vi "Abstract_Function_Hierarchy.vi"   [LabVIEW 2021]
uses:
  One Terminal/Boolean/AbsFunc_One Term_Bool.lvclass
  One Terminal/STR/AbsFunc_One Term_STR.lvclass
  One Terminal/SGL/AbsFunc_One Term_SGL.lvclass
  One Terminal/DBL/AbsFunc_One Term_DBL.lvclass
  One Terminal/EXT/AbsFunc_One Term_EXT.lvclass
  One Terminal/Cmplx SGL/AbsFunc_One Term_Complex SGL.lvclass
  One Terminal/Cmplx DBL/AbsFunc_One Term_Complex DBL.lvclass
  One Terminal/Cmplx EXT/AbsFunc_One Term_Complex EXT.lvclass
  One Terminal/I8/AbsFunc_One Term_I8.lvclass
  One Terminal/I16/AbsFunc_One Term_I16.lvclass
  One Terminal/I32/AbsFunc_One Term_I32.lvclass
  One Terminal/I64/AbsFunc_One Term_I64.lvclass
  One Terminal/U8/AbsFunc_One Term_U8.lvclass
  One Terminal/U16/AbsFunc_One Term_U16.lvclass
  One Terminal/U32/AbsFunc_One Term_U32.lvclass
  One Terminal/U64/AbsFunc_One Term_U64.lvclass
  One Terminal/Time/AbsFunc_One Term_Time.lvclass
  One Terminal/WFM_Numeric/AbsFunc_One Term_WFM_Numeric.lvclass
  Two Terminal/Boolean/AbsFunc_Two Term_Bool.lvclass
  Two Terminal/STR/AbsFunc_Two Term_STR.lvclass
  Two Terminal/SGL/AbsFunc_Two Term_SGL.lvclass
  Two Terminal/EXT/AbsFunc_Two Term_EXT.lvclass
  Two Terminal/DBL/AbsFunc_Two Term_DBL.lvclass
  Two Terminal/Cmplx SGL/AbsFunc_Two Term_Complex SGL.lvclass
  Two Terminal/Cmplx DBL/AbsFunc_Two Term_Complex DBL.lvclass
  Two Terminal/Cmplx EXT/AbsFunc_Two Term_Complex EXT.lvclass
  Two Terminal/I8/AbsFunc_Two Term_I8.lvclass
  Two Terminal/I16/AbsFunc_Two Term_I16.lvclass
  Two Terminal/I32/AbsFunc_Two Term_I32.lvclass
  Two Terminal/I64/AbsFunc_Two Term_I64.lvclass
  Two Terminal/U8/AbsFunc_Two Term_U8.lvclass
  Two Terminal/U16/AbsFunc_Two Term_U16.lvclass
  Two Terminal/U32/AbsFunc_Two Term_U32.lvclass
  Two Terminal/U64/AbsFunc_Two Term_U64.lvclass
  Two Terminal/Time/AbsFunc_Two Term_Time.lvclass
  Two Terminal/WFM_Numeric/AbsFunc_Two Term_WFM_Numeric.lvclass
  Abs_Types/Boolean/Abs_Boolean.lvclass
  Abs_Types/String/Abs_String.lvclass
  Abs_Types/Single Float/Abs_Single Float.lvclass
  Abs_Types/Double Float/Abs_Double Float.lvclass
  Abs_Types/Extended Float/Abs_Extended Float.lvclass
  Abs_Types/Complex Single Float/Abs_Complex Single Float.lvclass
  Abs_Types/Complex Double Float/Abs_Complex Double Float.lvclass
  Abs_Types/Complex Extended Float/Abs_Complex Extended Float.lvclass
  Abs_Types/I8 Integer/Abs_I8 Integer.lvclass
  Abs_Types/I16 Integer/Abs_I16 Integer.lvclass
  Abs_Types/I32 Integer/Abs_I32 Integer.lvclass
  Abs_Types/I64 Integer/Abs_I64 Integer.lvclass
  Abs_Types/U8 Integer/Abs_U8 Integer.lvclass
  Abs_Types/U16 Integer/Abs_U16 Integer.lvclass
  Abs_Types/U32 Integer/Abs_U32 Integer.lvclass
  Abs_Types/U64 Integer/Abs_U64 Integer.lvclass
  Abs_Types/Time/Abs_Time.lvclass
  Abs_Types/Waveform/Abs_Waveform.lvclass
panel:
  # "SEE DIAGRAM\nFOR Hierarchy"
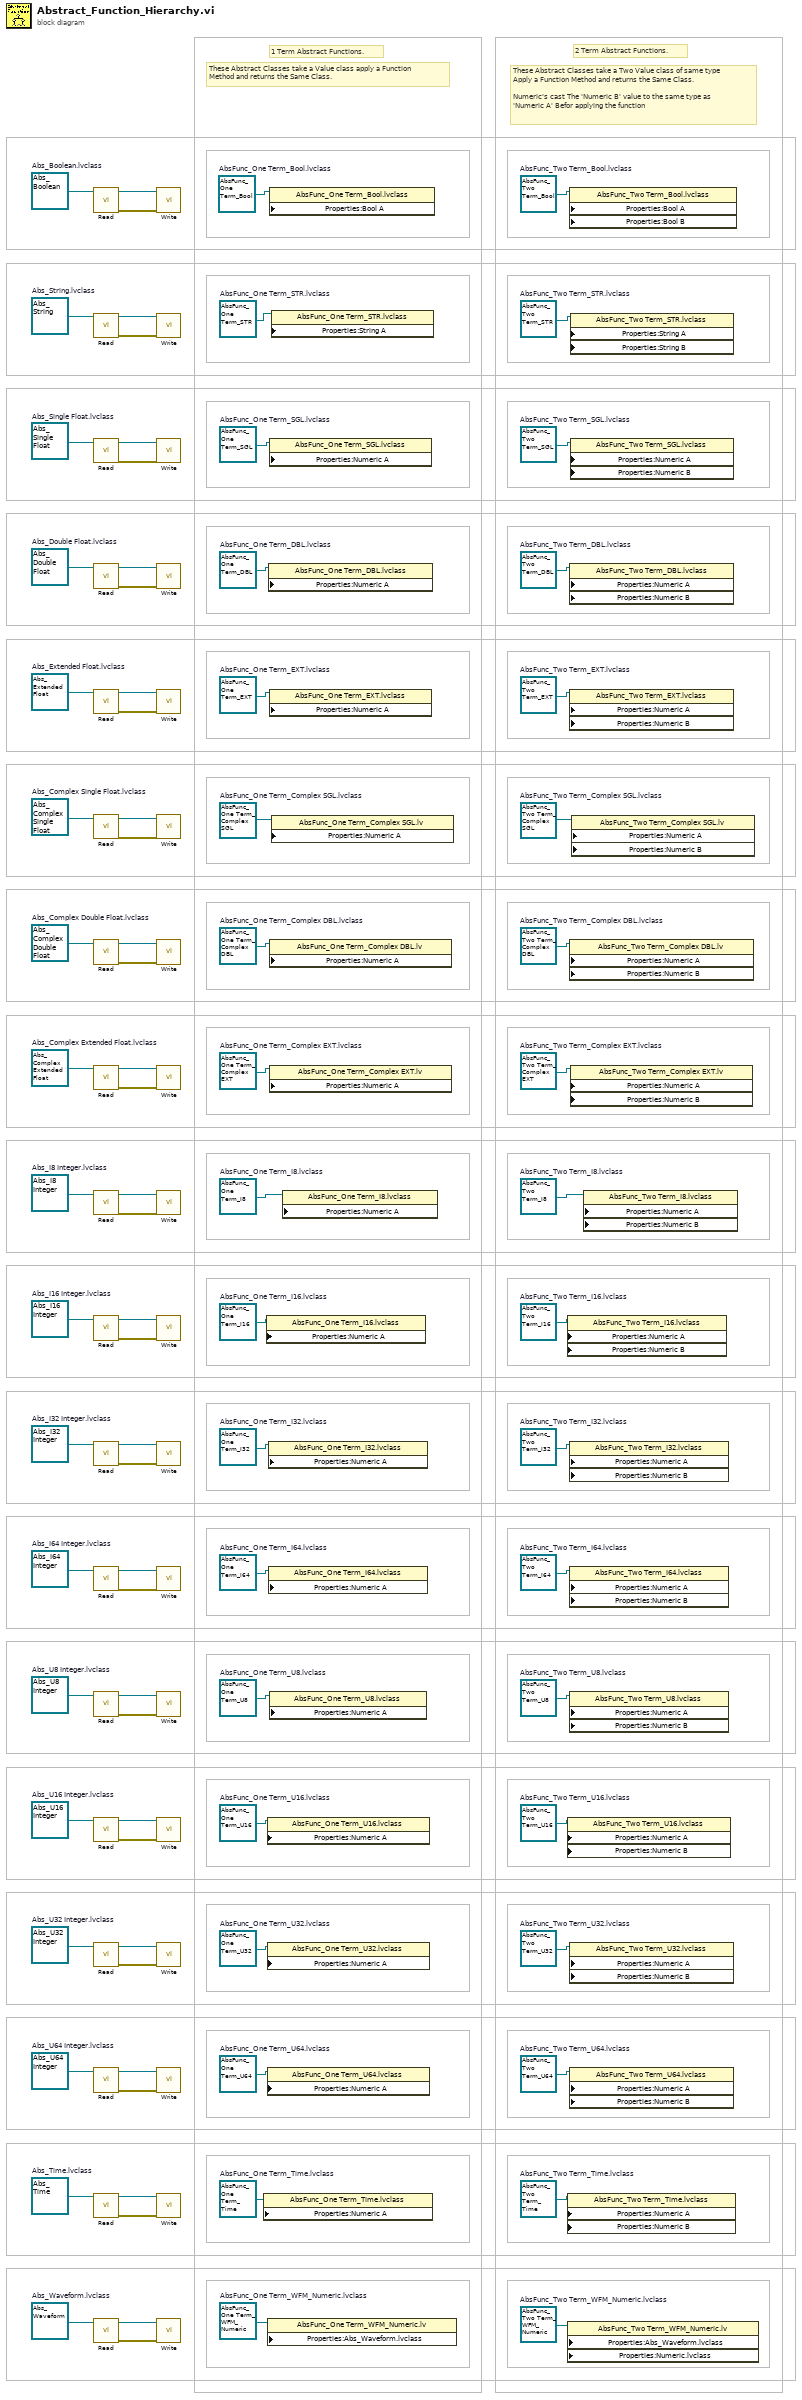
[diagram p0: block diagram]
diagram:
  w2 = refnum<class "Abs_Waveform.lvclass"> refnum  # Abs_Waveform.lvclass
  w7 = refnum<class "Abs_Time.lvclass"> refnum  # Abs_Time.lvclass
  w8 = refnum<class "Abs_U64 Integer.lvclass"> refnum  # Abs_U64 Integer.lvclass
  w11 = refnum<class "Abs_U32 Integer.lvclass"> refnum  # Abs_U32 Integer.lvclass
  w14 = refnum<class "Abs_U16 Integer.lvclass"> refnum  # Abs_U16 Integer.lvclass
  w17 = refnum<class "Abs_U8 Integer.lvclass"> refnum  # Abs_U8 Integer.lvclass
  w22 = refnum<class "Abs_I64 Integer.lvclass"> refnum  # Abs_I64 Integer.lvclass
  w23 = refnum<class "Abs_I32 Integer.lvclass"> refnum  # Abs_I32 Integer.lvclass
  w26 = refnum<class "Abs_I16 Integer.lvclass"> refnum  # Abs_I16 Integer.lvclass
  w29 = refnum<class "Abs_I8 Integer.lvclass"> refnum  # Abs_I8 Integer.lvclass
  w32 = refnum<class "Abs_Complex Extended Float.lvclass"> refnum  # Abs_Complex Extended Float.lvclass
  w35 = refnum<class "Abs_Complex Double Float.lvclass"> refnum  # Abs_Complex Double Float.lvclass
  w38 = refnum<class "Abs_Complex Single Float.lvclass"> refnum  # Abs_Complex Single Float.lvclass
  w41 = refnum<class "Abs_Extended Float.lvclass"> refnum  # Abs_Extended Float.lvclass
  w44 = refnum<class "Abs_Double Float.lvclass"> refnum  # Abs_Double Float.lvclass
  w47 = refnum<class "Abs_Single Float.lvclass"> refnum  # Abs_Single Float.lvclass
  w50 = refnum<class "Abs_String.lvclass"> refnum  # Abs_String.lvclass
  w55 = refnum<class "Abs_Boolean.lvclass"> refnum  # Abs_Boolean.lvclass
  w63 = refnum<class "AbsFunc_Two Term_WFM_Numeric.lvclass"> refnum  # AbsFunc_Two Term_WFM_Numeric.lvclass
  w64 = refnum<class "AbsFunc_Two Term_Time.lvclass"> refnum  # AbsFunc_Two Term_Time.lvclass
  w65 = refnum<class "AbsFunc_Two Term_U64.lvclass"> refnum  # AbsFunc_Two Term_U64.lvclass
  w66 = refnum<class "AbsFunc_Two Term_U32.lvclass"> refnum  # AbsFunc_Two Term_U32.lvclass
  w67 = refnum<class "AbsFunc_Two Term_U16.lvclass"> refnum  # AbsFunc_Two Term_U16.lvclass
  w68 = refnum<class "AbsFunc_Two Term_U8.lvclass"> refnum  # AbsFunc_Two Term_U8.lvclass
  w69 = refnum<class "AbsFunc_Two Term_I64.lvclass"> refnum  # AbsFunc_Two Term_I64.lvclass
  w70 = refnum<class "AbsFunc_Two Term_I32.lvclass"> refnum  # AbsFunc_Two Term_I32.lvclass
  w71 = refnum<class "AbsFunc_Two Term_I16.lvclass"> refnum  # AbsFunc_Two Term_I16.lvclass
  w72 = refnum<class "AbsFunc_Two Term_I8.lvclass"> refnum  # AbsFunc_Two Term_I8.lvclass
  w73 = refnum<class "AbsFunc_Two Term_Complex EXT.lvclass"> refnum  # AbsFunc_Two Term_Complex EXT.lvclass
  w74 = refnum<class "AbsFunc_Two Term_Complex DBL.lvclass"> refnum  # AbsFunc_Two Term_Complex DBL.lvclass
  w75 = refnum<class "AbsFunc_Two Term_Complex SGL.lvclass"> refnum  # AbsFunc_Two Term_Complex SGL.lvclass
  w77 = refnum<class "AbsFunc_Two Term_DBL.lvclass"> refnum  # AbsFunc_Two Term_DBL.lvclass
  w76 = refnum<class "AbsFunc_Two Term_EXT.lvclass"> refnum  # AbsFunc_Two Term_EXT.lvclass
  w78 = refnum<class "AbsFunc_Two Term_SGL.lvclass"> refnum  # AbsFunc_Two Term_SGL.lvclass
  w79 = refnum<class "AbsFunc_Two Term_STR.lvclass"> refnum  # AbsFunc_Two Term_STR.lvclass
  w80 = refnum<class "AbsFunc_Two Term_Bool.lvclass"> refnum  # AbsFunc_Two Term_Bool.lvclass
  w62 = refnum<class "AbsFunc_One Term_WFM_Numeric.lvclass"> refnum  # AbsFunc_One Term_WFM_Numeric.lvclass
  w61 = refnum<class "AbsFunc_One Term_Time.lvclass"> refnum  # AbsFunc_One Term_Time.lvclass
  w60 = refnum<class "AbsFunc_One Term_U64.lvclass"> refnum  # AbsFunc_One Term_U64.lvclass
  w59 = refnum<class "AbsFunc_One Term_U32.lvclass"> refnum  # AbsFunc_One Term_U32.lvclass
  w1 = refnum<class "AbsFunc_One Term_U16.lvclass"> refnum  # AbsFunc_One Term_U16.lvclass
  w58 = refnum<class "AbsFunc_One Term_U8.lvclass"> refnum  # AbsFunc_One Term_U8.lvclass
  w57 = refnum<class "AbsFunc_One Term_I64.lvclass"> refnum  # AbsFunc_One Term_I64.lvclass
  w56 = refnum<class "AbsFunc_One Term_I32.lvclass"> refnum  # AbsFunc_One Term_I32.lvclass
  w81 = refnum<class "AbsFunc_One Term_I16.lvclass"> refnum  # AbsFunc_One Term_I16.lvclass
  w82 = refnum<class "AbsFunc_One Term_I8.lvclass"> refnum  # AbsFunc_One Term_I8.lvclass
  w83 = refnum<class "AbsFunc_One Term_Complex EXT.lvclass"> refnum  # AbsFunc_One Term_Complex EXT.lvclass
  w84 = refnum<class "AbsFunc_One Term_Complex DBL.lvclass"> refnum  # AbsFunc_One Term_Complex DBL.lvclass
  w85 = refnum<class "AbsFunc_One Term_Complex SGL.lvclass"> refnum  # AbsFunc_One Term_Complex SGL.lvclass
  w86 = refnum<class "AbsFunc_One Term_EXT.lvclass"> refnum  # AbsFunc_One Term_EXT.lvclass
  w87 = refnum<class "AbsFunc_One Term_DBL.lvclass"> refnum  # AbsFunc_One Term_DBL.lvclass
  w88 = refnum<class "AbsFunc_One Term_SGL.lvclass"> refnum  # AbsFunc_One Term_SGL.lvclass
  w89 = refnum<class "AbsFunc_One Term_STR.lvclass"> refnum  # AbsFunc_One Term_STR.lvclass
  w90 = refnum<class "AbsFunc_One Term_Bool.lvclass"> refnum  # AbsFunc_One Term_Bool.lvclass
  # "1 Term Abstract Functions."
  # "These Abstract Classes take a Value class apply a Function \nMethod and returns the Same Class."
  # "These Abstract Classes take a Two Value class of same type\nApply a Function Method and returns the Same Class.\n\nNumeric's cast The 'Numeric B' value to the same type as \n'Numeric A' Befor applying the function"
  # "2 Term Abstract Functions."
  n1 = call-dynamic "Read.vi"("Boolean in"=w55) -> ("error out"=w54:errorcluster, "Boolean out"=w53:refnum<class "Abs_Boolean.lvclass">)  [unwired: 8 in, 1 out]
  n2 = call-dynamic "Read.vi"("Abs_String in"=w50) -> ("error out"=w52:errorcluster, "Abs_String out"=w51:refnum<class "Abs_String.lvclass">)  [unwired: 8 in, 1 out]
  n3 = call-dynamic "Read.vi"("Double Float.lvclass_340760 in"=w47) -> ("error out"=w49:errorcluster, "Double Float.lvclass_340760 out"=w48:refnum<class "Abs_Single Float.lvclass">)  [unwired: 8 in, 1 out]
  n4 = call-dynamic "Read.vi"("Double Float.lvclass_340760 in"=w44) -> ("error out"=w46:errorcluster, "Double Float.lvclass_340760 out"=w45:refnum<class "Abs_Double Float.lvclass">)  [unwired: 8 in, 1 out]
  n5 = call-dynamic "Read.vi"("Double Float.lvclass_340760 in"=w41) -> ("error out"=w43:errorcluster, "Double Float.lvclass_340760 out"=w42:refnum<class "Abs_Extended Float.lvclass">)  [unwired: 8 in, 1 out]
  n6 = call-dynamic "Read.vi"("Double Float.lvclass_340760 in"=w38) -> ("error out"=w40:errorcluster, "Double Float.lvclass_340760 out"=w39:refnum<class "Abs_Complex Single Float.lvclass">)  [unwired: 8 in, 1 out]
  n7 = call-dynamic "Read.vi"("Double Float.lvclass_340760 in"=w35) -> ("error out"=w37:errorcluster, "Double Float.lvclass_340760 out"=w36:refnum<class "Abs_Complex Double Float.lvclass">)  [unwired: 8 in, 1 out]
  n8 = call-dynamic "Read.vi"("Double Float.lvclass_340760 in"=w32) -> ("error out"=w34:errorcluster, "Double Float.lvclass_340760 out"=w33:refnum<class "Abs_Complex Extended Float.lvclass">)  [unwired: 8 in, 1 out]
  n9 = call-dynamic "Read.vi"("Double Float.lvclass_340760 in"=w29) -> ("error out"=w31:errorcluster, "Double Float.lvclass_340760 out"=w30:refnum<class "Abs_I8 Integer.lvclass">)  [unwired: 8 in, 1 out]
  n10 = call-dynamic "Read.vi"("Double Float.lvclass_340760 in"=w26) -> ("error out"=w28:errorcluster, "Double Float.lvclass_340760 out"=w27:refnum<class "Abs_I16 Integer.lvclass">)  [unwired: 8 in, 1 out]
  n11 = call-dynamic "Read.vi"("Double Float.lvclass_340760 in"=w23) -> ("error out"=w25:errorcluster, "Double Float.lvclass_340760 out"=w24:refnum<class "Abs_I32 Integer.lvclass">)  [unwired: 8 in, 1 out]
  n12 = call-dynamic "Read.vi"("Double Float.lvclass_340760 in"=w22) -> ("error out"=w21:errorcluster, "Double Float.lvclass_340760 out"=w20:refnum<class "Abs_I64 Integer.lvclass">)  [unwired: 8 in, 1 out]
  n13 = call-dynamic "Read.vi"("Double Float.lvclass_340760 in"=w17) -> ("error out"=w19:errorcluster, "Double Float.lvclass_340760 out"=w18:refnum<class "Abs_U8 Integer.lvclass">)  [unwired: 8 in, 1 out]
  n14 = call-dynamic "Read.vi"("Double Float.lvclass_340760 in"=w14) -> ("error out"=w16:errorcluster, "Double Float.lvclass_340760 out"=w15:refnum<class "Abs_U16 Integer.lvclass">)  [unwired: 8 in, 1 out]
  n15 = call-dynamic "Read.vi"("Double Float.lvclass_340760 in"=w11) -> ("error out"=w13:errorcluster, "Double Float.lvclass_340760 out"=w12:refnum<class "Abs_U32 Integer.lvclass">)  [unwired: 8 in, 1 out]
  n16 = call-dynamic "Read.vi"("Double Float.lvclass_340760 in"=w8) -> ("error out"=w10:errorcluster, "Double Float.lvclass_340760 out"=w9:refnum<class "Abs_U64 Integer.lvclass">)  [unwired: 8 in, 1 out]
  n17 = call-dynamic "Read.vi"("Double Float.lvclass_340760 in"=w7) -> ("error out"=w5:errorcluster, "Double Float.lvclass_340760 out"=w6:refnum<class "Abs_Time.lvclass">)  [unwired: 8 in, 1 out]
  n18 = call-dynamic "Read.vi"("Abs_Waveform in"=w2) -> ("error out"=w3:errorcluster, "Abs_Waveform out"=w4:refnum<class "Abs_Waveform.lvclass">)  [unwired: 8 in, 1 out]
  n19 = call-dynamic "Write.vi"("error in (no error)"=w54, "Boolean in"=w53) -> ()  [unwired: 8 in, 2 out]
  n20 = call-dynamic "Write.vi"("error in (no error)"=w52, "Abs_String in"=w51) -> ()  [unwired: 8 in, 2 out]
  n21 = call-dynamic "Write.vi"("error in (no error)"=w49, "Double Float.lvclass_340760 in"=w48) -> ()  [unwired: 8 in, 2 out]
  n22 = call-dynamic "Write.vi"("error in (no error)"=w46, "Double Float.lvclass in"=w45) -> ()  [unwired: 8 in, 2 out]
  n23 = call-dynamic "Write.vi"("error in (no error)"=w43, "Double Float.lvclass_340760 in"=w42) -> ()  [unwired: 8 in, 2 out]
  n24 = call-dynamic "Write.vi"("error in (no error)"=w40, "Double Float.lvclass_340760 in"=w39) -> ()  [unwired: 8 in, 2 out]
  n25 = call-dynamic "Write.vi"("error in (no error)"=w37, "Double Float.lvclass_340760 in"=w36) -> ()  [unwired: 8 in, 2 out]
  n26 = call-dynamic "Write.vi"("error in (no error)"=w34, "Double Float.lvclass_340760 in"=w33) -> ()  [unwired: 8 in, 2 out]
  n27 = call-dynamic "Write.vi"("error in (no error)"=w31, "Double Float.lvclass_340760 in"=w30) -> ()  [unwired: 8 in, 2 out]
  n28 = call-dynamic "Write.vi"("error in (no error)"=w28, "Double Float.lvclass_340760 in"=w27) -> ()  [unwired: 8 in, 2 out]
  n29 = call-dynamic "Write.vi"("error in (no error)"=w25, "Double Float.lvclass_340760 in"=w24) -> ()  [unwired: 8 in, 2 out]
  n30 = call-dynamic "Write.vi"("error in (no error)"=w21, "Double Float.lvclass_340760 in"=w20) -> ()  [unwired: 8 in, 2 out]
  n31 = call-dynamic "Write.vi"("error in (no error)"=w19, "Double Float.lvclass_340760 in"=w18) -> ()  [unwired: 8 in, 2 out]
  n32 = call-dynamic "Write.vi"("error in (no error)"=w16, "Double Float.lvclass_340760 in"=w15) -> ()  [unwired: 8 in, 2 out]
  n33 = call-dynamic "Write.vi"("error in (no error)"=w13, "Double Float.lvclass_340760 in"=w12) -> ()  [unwired: 8 in, 2 out]
  n34 = call-dynamic "Write.vi"("error in (no error)"=w10, "Double Float.lvclass_340760 in"=w9) -> ()  [unwired: 8 in, 2 out]
  n35 = call-dynamic "Write.vi"("error in (no error)"=w5, "Double Float.lvclass_340760 in"=w6) -> ()  [unwired: 8 in, 2 out]
  n36 = call-dynamic "Write.vi"("error in (no error)"=w3, "Abs_Waveform in"=w4) -> ()  [unwired: 8 in, 2 out]
  n37 = property class="AbsFunc_One Term_Time.lvclass" props=["Properties:Numeric A"](reference=w61) -> ()  [unwired: 2 in, 2 out]
  n38 = property class="AbsFunc_One Term_I16.lvclass" props=["Properties:Numeric A"](reference=w81) -> ()  [unwired: 2 in, 2 out]
  n39 = property class="AbsFunc_One Term_U16.lvclass" props=["Properties:Numeric A"](reference=w1) -> ()  [unwired: 2 in, 2 out]
  n40 = property class="AbsFunc_One Term_U32.lvclass" props=["Properties:Numeric A"](reference=w59) -> ()  [unwired: 2 in, 2 out]
  n41 = property class="AbsFunc_One Term_U64.lvclass" props=["Properties:Numeric A"](reference=w60) -> ()  [unwired: 2 in, 2 out]
  n42 = property class="AbsFunc_One Term_WFM_Numeric.lv" props=["Properties:Abs_Waveform.lvclass"](reference=w62) -> ()  [unwired: 2 in, 2 out]
  n43 = property class="AbsFunc_One Term_DBL.lvclass" props=["Properties:Numeric A"](reference=w87) -> ()  [unwired: 2 in, 2 out]
  n44 = property class="AbsFunc_One Term_I32.lvclass" props=["Properties:Numeric A"](reference=w56) -> ()  [unwired: 2 in, 2 out]
  n45 = property class="AbsFunc_One Term_I64.lvclass" props=["Properties:Numeric A"](reference=w57) -> ()  [unwired: 2 in, 2 out]
  n46 = property class="AbsFunc_One Term_Bool.lvclass" props=["Properties:Bool A"](reference=w90) -> ()  [unwired: 2 in, 2 out]
  n47 = property class="AbsFunc_One Term_SGL.lvclass" props=["Properties:Numeric A"](reference=w88) -> ()  [unwired: 2 in, 2 out]
  n48 = property class="AbsFunc_One Term_EXT.lvclass" props=["Properties:Numeric A"](reference=w86) -> ()  [unwired: 2 in, 2 out]
  n49 = property class="AbsFunc_One Term_Complex DBL.lv" props=["Properties:Numeric A"](reference=w84) -> ()  [unwired: 2 in, 2 out]
  n50 = property class="AbsFunc_One Term_Complex EXT.lv" props=["Properties:Numeric A"](reference=w83) -> ()  [unwired: 2 in, 2 out]
  n51 = property class="AbsFunc_One Term_U8.lvclass" props=["Properties:Numeric A"](reference=w58) -> ()  [unwired: 2 in, 2 out]
  n52 = property class="AbsFunc_One Term_STR.lvclass" props=["Properties:String A"](reference=w89) -> ()  [unwired: 2 in, 2 out]
  n53 = property class="AbsFunc_One Term_Complex SGL.lv" props=["Properties:Numeric A"](reference=w85) -> ()  [unwired: 2 in, 2 out]
  n54 = property class="AbsFunc_One Term_I8.lvclass" props=["Properties:Numeric A"](reference=w82) -> ()  [unwired: 2 in, 2 out]
  n55 = property class="AbsFunc_Two Term_I16.lvclass" props=["Properties:Numeric A", "Properties:Numeric B"](reference=w71) -> ()  [unwired: 3 in, 2 out]
  n56 = property class="AbsFunc_Two Term_U16.lvclass" props=["Properties:Numeric A", "Properties:Numeric B"](reference=w67) -> ()  [unwired: 3 in, 2 out]
  n57 = property class="AbsFunc_Two Term_Time.lvclass" props=["Properties:Numeric A", "Properties:Numeric B"](reference=w64) -> ()  [unwired: 3 in, 2 out]
  n58 = property class="AbsFunc_Two Term_WFM_Numeric.lv" props=["Properties:Abs_Waveform.lvclass", "Properties:Numeric.lvclass"](reference=w63) -> ()  [unwired: 3 in, 2 out]
  n59 = property class="AbsFunc_Two Term_Bool.lvclass" props=["Properties:Bool A", "Properties:Bool B"](reference=w80) -> ()  [unwired: 3 in, 2 out]
  n60 = property class="AbsFunc_Two Term_DBL.lvclass" props=["Properties:Numeric A", "Properties:Numeric B"](reference=w77) -> ()  [unwired: 3 in, 2 out]
  n61 = property class="AbsFunc_Two Term_EXT.lvclass" props=["Properties:Numeric A", "Properties:Numeric B"](reference=w76) -> ()  [unwired: 3 in, 2 out]
  n62 = property class="AbsFunc_Two Term_Complex DBL.lv" props=["Properties:Numeric A", "Properties:Numeric B"](reference=w74) -> ()  [unwired: 3 in, 2 out]
  n63 = property class="AbsFunc_Two Term_I32.lvclass" props=["Properties:Numeric A", "Properties:Numeric B"](reference=w70) -> ()  [unwired: 3 in, 2 out]
  n64 = property class="AbsFunc_Two Term_I64.lvclass" props=["Properties:Numeric A", "Properties:Numeric B"](reference=w69) -> ()  [unwired: 3 in, 2 out]
  n65 = property class="AbsFunc_Two Term_U8.lvclass" props=["Properties:Numeric A", "Properties:Numeric B"](reference=w68) -> ()  [unwired: 3 in, 2 out]
  n66 = property class="AbsFunc_Two Term_U32.lvclass" props=["Properties:Numeric A", "Properties:Numeric B"](reference=w66) -> ()  [unwired: 3 in, 2 out]
  n67 = property class="AbsFunc_Two Term_U64.lvclass" props=["Properties:Numeric A", "Properties:Numeric B"](reference=w65) -> ()  [unwired: 3 in, 2 out]
  n68 = property class="AbsFunc_Two Term_STR.lvclass" props=["Properties:String A", "Properties:String B"](reference=w79) -> ()  [unwired: 3 in, 2 out]
  n69 = property class="AbsFunc_Two Term_SGL.lvclass" props=["Properties:Numeric A", "Properties:Numeric B"](reference=w78) -> ()  [unwired: 3 in, 2 out]
  n70 = property class="AbsFunc_Two Term_Complex EXT.lv" props=["Properties:Numeric A", "Properties:Numeric B"](reference=w73) -> ()  [unwired: 3 in, 2 out]
  n71 = property class="AbsFunc_Two Term_Complex SGL.lv" props=["Properties:Numeric A", "Properties:Numeric B"](reference=w75) -> ()  [unwired: 3 in, 2 out]
  n72 = property class="AbsFunc_Two Term_I8.lvclass" props=["Properties:Numeric A", "Properties:Numeric B"](reference=w72) -> ()  [unwired: 3 in, 2 out]
